vi "Main Page.vi"(8 "error in (no error)":errorcluster, 11 "Node Ptr":T7 format="%.0x") -> (0 "error out":errorcluster)   [LabVIEW 2020, in "Modbus Master System Explorer.lvlib"]
uses:
  Modbus Master System Explorer.lvlib
  <vilib>/NI VeriStand/Custom Device API/Custom Device Item Ref.ctl
  Shared/Controls/Interface Type.ctl
  Shared/Controls/Parity.ctl
  Shared/Controls/Serial Type.ctl
  Shared/Controls/Flow Control.ctl
  SubVIs/Radix.ctl
  Shared/Write Mode.ctl
  Shared/Constants.vi
  <vilib>/NI VeriStand/Custom Device API/Set Item Property (U16).vi
  <vilib>/NI VeriStand/Custom Device API/Custom Device API.lvlib
  Shared/Modbus Master Shared.lvlib
panel:
  out "Version":string
  in  "Write Refresh Rate (ms)":i32
  in  "Write Mode":T1
  in  "WebBrowser":refnum<k7>(container)
  in  "Maximum Channels per Read":i32
  in  "Read Refresh Rate (ms)":i32
  in  "Export to Kepware Server":bool
  in  "Name":string
  in  "Master Settings Tabs":enum32{"TCP Master", "Serial Master"}(tab)
  in  "Timeout (ms)":i32
  in  "Address":string
  in  "Port":u16
  in  "Baud Rate":string(combo)
  in  "Radix":T2
  in  "Unit ID":u16
  out "Data Bits":u32=7
  in  "VISA resource name":refnum<visa-resource-name>
  in  "flow control (none)":T3 items=["None", "XON/XOFF", "RTS/CTS", "XON/XOFF & RTS/CTS", "DTR/DSR", "XON/XOFF & DTR/DSR"]
  in  "parity (even)":T4=2 items=["None", "Odd", "Even", "Mark", "Space"]
  in  "serial type":T5
  out "Stop Bits":u32
  in  "Wire Mode":i16(ring)=-1 items=["Unknown"=-1, "RS485/Wire4"=0, "RS485/Wire2-EchoDTR"=1, "RS485/Wire2-CtrlDTR"=2, "RS485/Wire2-Auto"=3, "RS232/DTE"=128, "RS232/DCE"=129, "RS232/AUTO"=130]
  in  "Interface Type":T6
  in  "Header":cluster{"Section Name":string}={"Section Name"="Modbus Master to Slave Settings"}
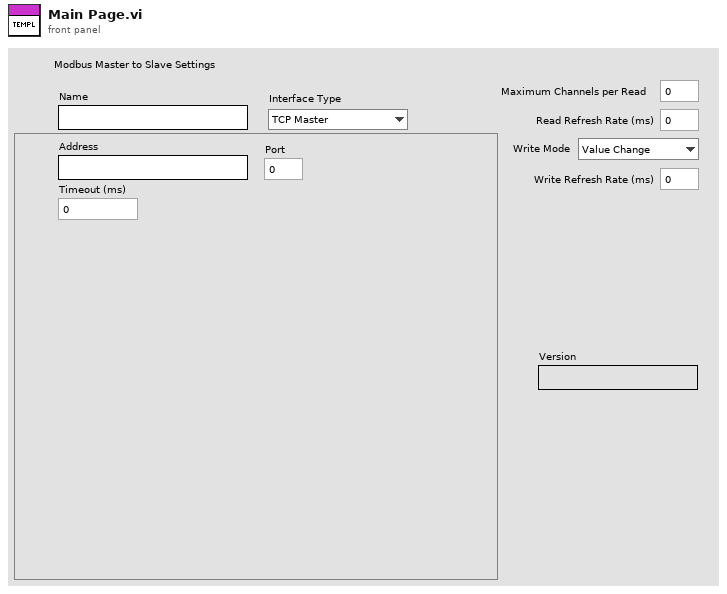
[diagram p1: front panel]
types:
  T1 = typedef "Modbus Master Shared.lvlib/Write Mode.ctl" = enum16{"Value Change", "Interval"}
  T2 = typedef "Modbus Master System Explorer.lvlib/Radix.ctl" = enum32{"Decimal", "Hexidecimal"}
  T3 = typedef "Modbus Master Shared.lvlib/Flow Control.ctl" = u16
  T4 = typedef "Modbus Master Shared.lvlib/Parity.ctl" = u16
  T5 = typedef "Modbus Master Shared.lvlib/Serial Type.ctl" = enum16{"RTU", "ASCII"}
  T6 = typedef "Modbus Master Shared.lvlib/Interface Type.ctl" = enum16{"TCP Master", "Serial Master", "TCP Slave", "Serial Slave"}
  T7 = typedef "Custom Device API.lvlib/Custom Device Item Ref.ctl" = u64
  T8 = enum8{"Enabled", "Disabled", "Disabled and Grayed Out"}
  T9 = typedef "Custom Device API.lvlib/Custom Device Commands.ctl" = enum16{"Default", "Item renamed", "Shutdown", "Dynamic button pressed"}
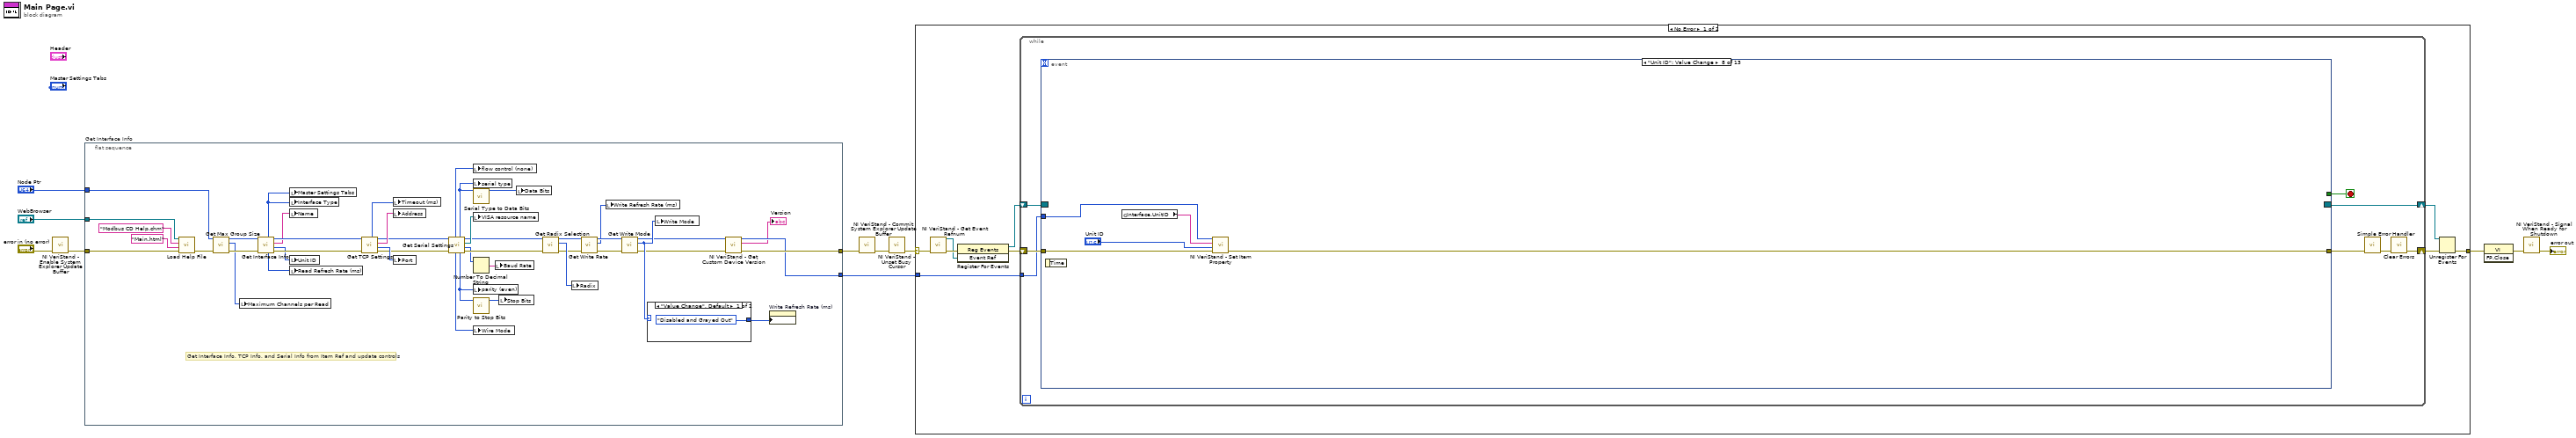
[diagram p0: block diagram]
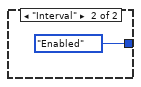
[diagram p2: hidden frame]
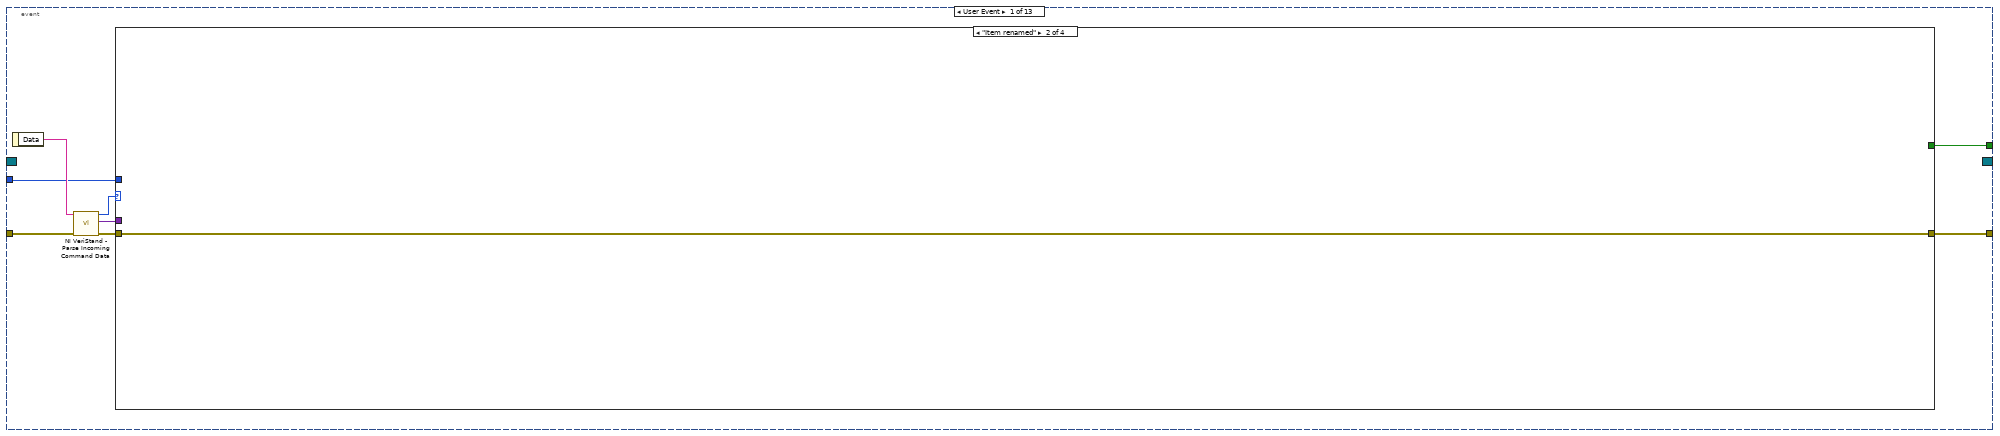
[diagram p3: hidden frame]
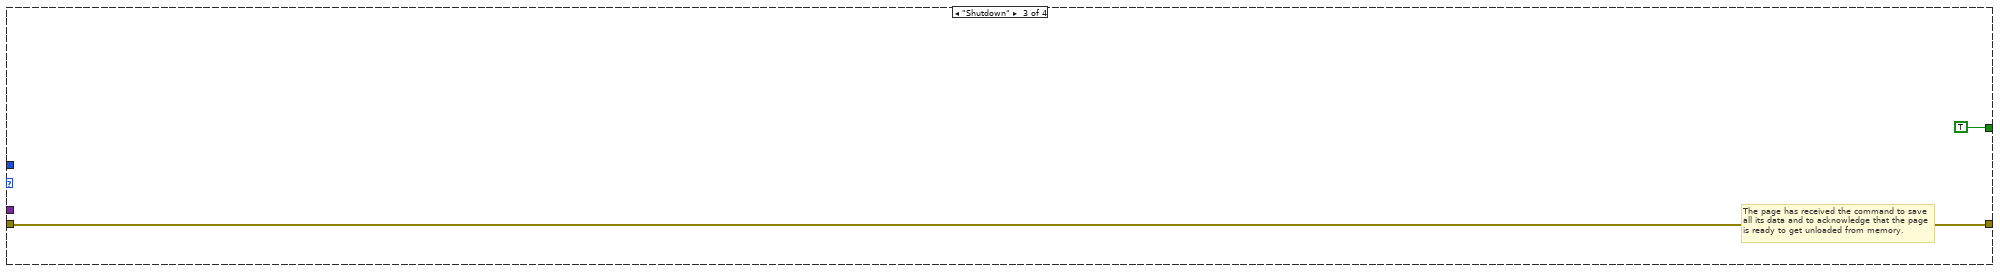
[diagram p5: hidden frame]
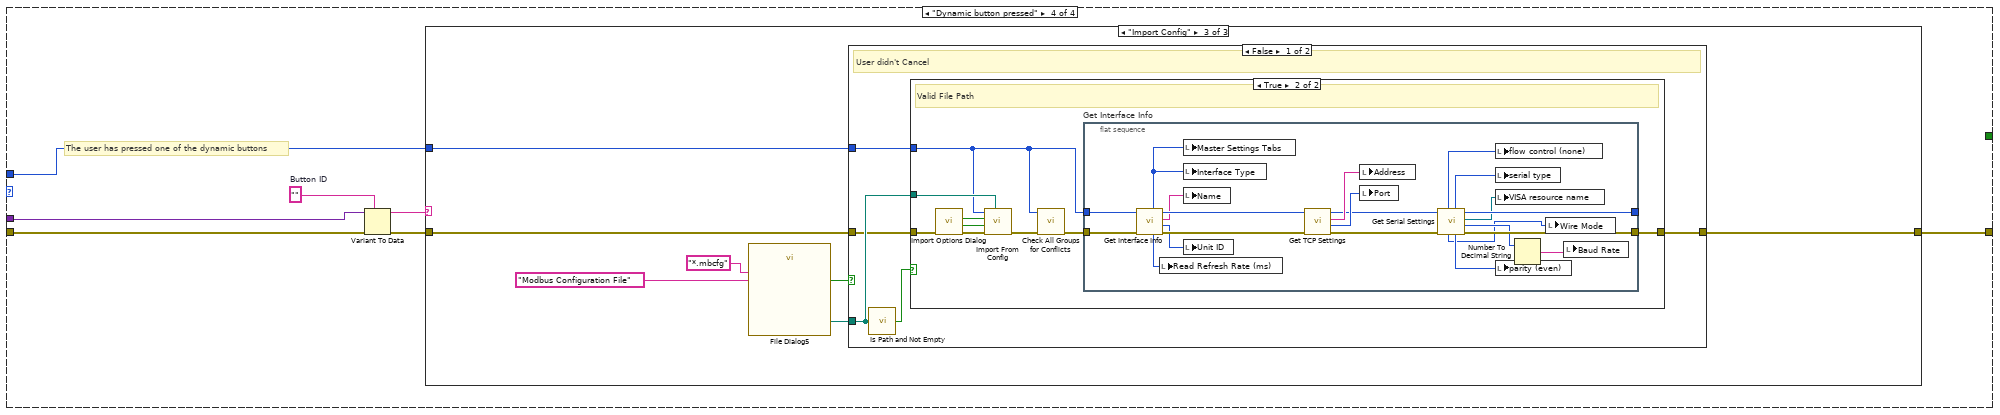
[diagram p6: hidden frame]
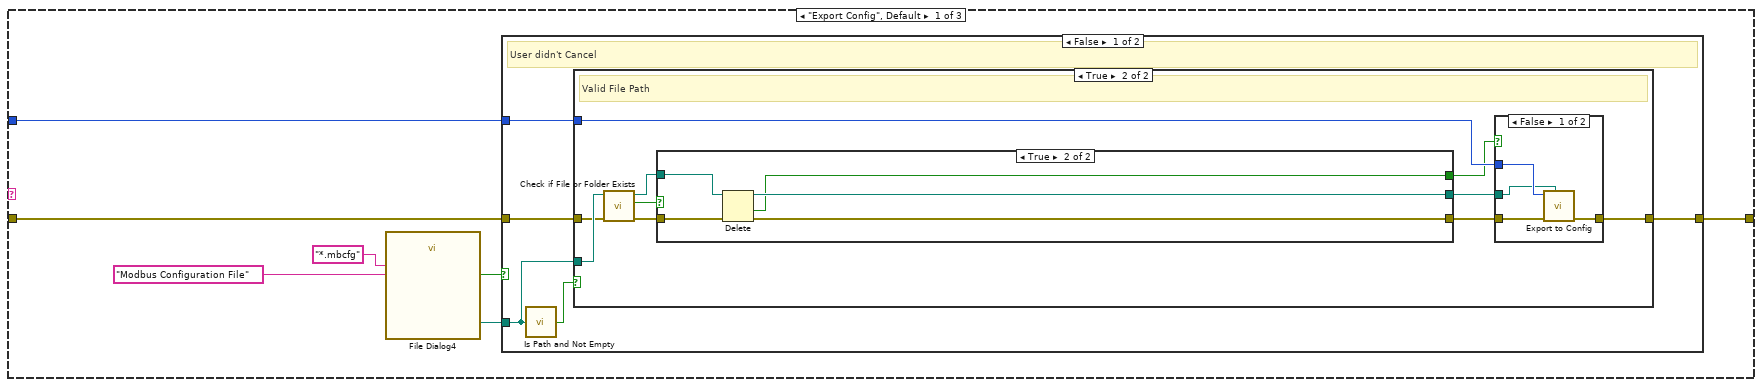
[diagram p7: hidden frame]
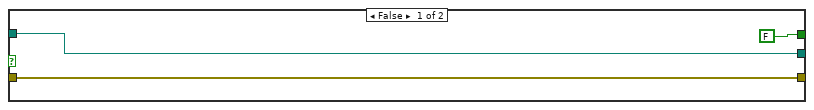
[diagram p9: hidden frame]
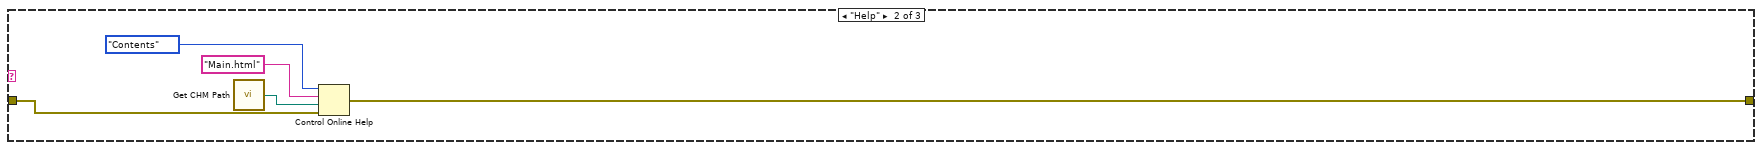
[diagram p12: hidden frame]
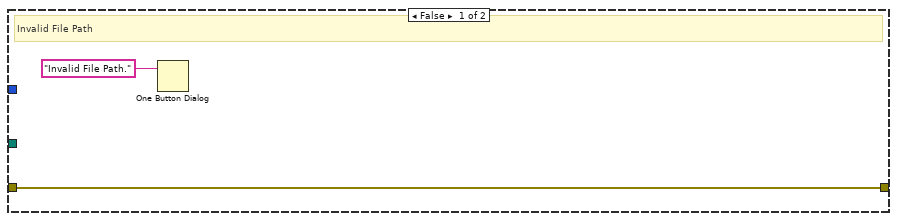
[diagram p13: hidden frame]
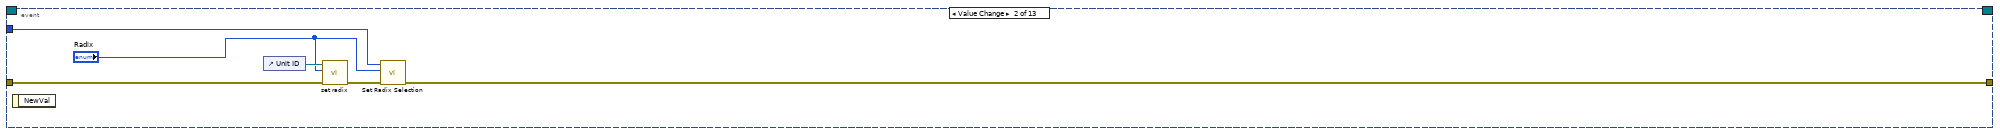
[diagram p15: hidden frame]
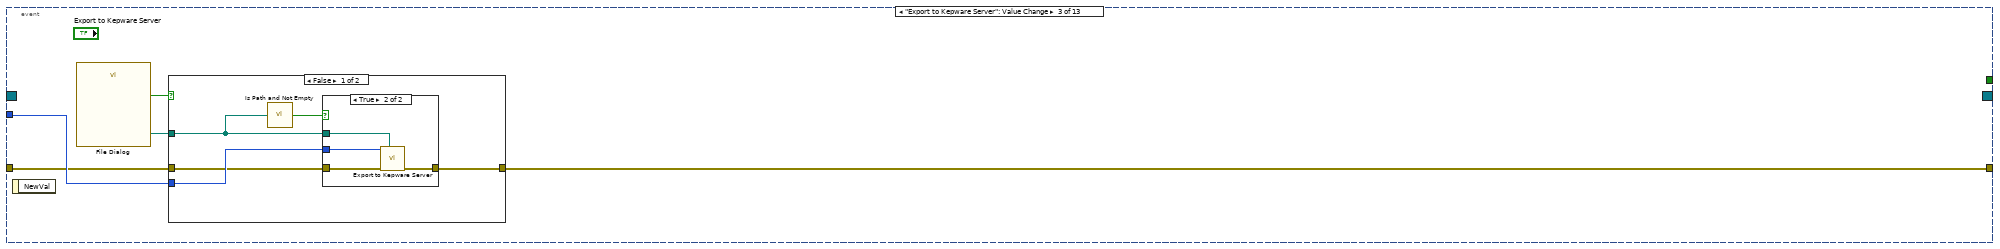
[diagram p16: hidden frame]
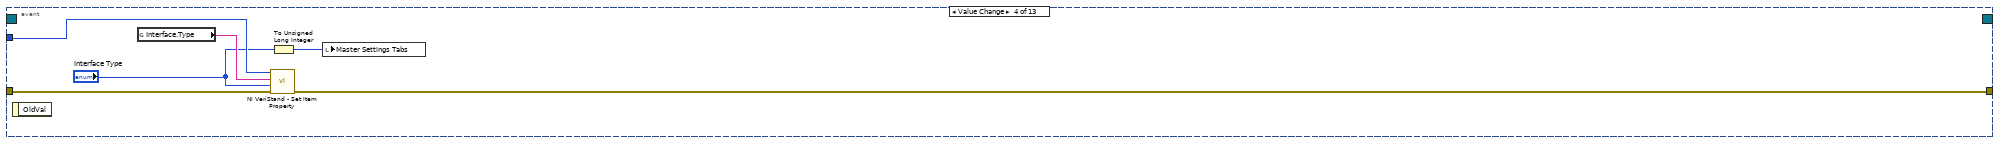
[diagram p19: hidden frame]
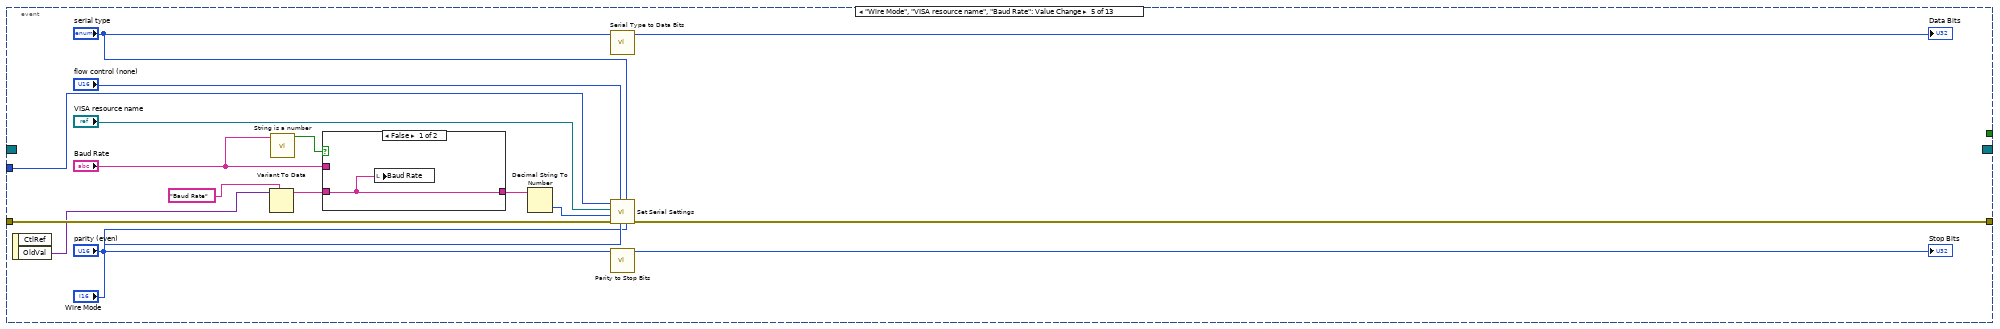
[diagram p20: hidden frame]
diagram:
  n1 = call <vilib>:"NI VeriStand - Enable System Explorer Update Buffer.vi"("error in (no error)"="error in (no error)") -> ("error out"=w1:errorcluster)  [unwired: 10 in]
  n2 = flat-sequence "Get Interface Info" {
    tunnel: w1 -> [w26]
    tunnel: "Node Ptr" -> [w39]
    tunnel: [w15] -> w4
    tunnel: [w13] -> w6
    tunnel: "WebBrowser" -> [w29]
    frame #0 {
      # "Get Interface Info, TCP Info, and Serial Info from Item Ref and update controls"
      n3 = call "Load Help File.vi"("error in (no error)"=w26, "HTML File"="Main.html", "Main CHM File"="Modbus CD Help.chm", "SHDocVw.IWebBrowser2"=w29) -> ("error out"=w25:errorcluster)  [unwired: 7 in]
      n4 = call "Get Max Group Size.vi"("error in (no error)"=w25, "Item Ref in"=w39) -> ("error out"=w37:errorcluster, "Value"=w36:i32, "Item Ref out"=w38:T7)  [unwired: 7 in]
      n5 = local write "Maximum Channels per Read"(w36) -> ()
      n6 = call "Get Interface Info.vi"("error in (no error)"=w37, "Device Item Ref in"=w38) -> ("error out"=w48:errorcluster, "Unit ID"=w45:u16, "Name"=w46:string, "Item Ref out"=w49:T7, "Refresh Rate"=w44:i32, "Interface Type"=w47:T6)  [unwired: 4 in]
      n7 = local write "Master Settings Tabs"(w47) -> ()
      n8 = local write "Interface Type"(w47) -> ()
      n9 = local write "Name"(w46) -> ()
      n10 = local write "Unit ID"(w45) -> ()
      n11 = local write "Read Refresh Rate (ms)"(w44) -> ()
      n12 = call "Get TCP Settings.vi"("error in (no error)"=w48, "Item Ref in"=w49) -> ("error out"=w53:errorcluster, "Port"=w54:u16, "Address"=w55:string, "Item Ref out"=w52:T7, "Timeout"=w35:i32)  [unwired: 5 in]
      n13 = local write "Timeout (ms)"(w35) -> ()
      n14 = local write "Address"(w55) -> ()
      n15 = local write "Port"(w54) -> ()
      n16 = call "Get Serial Settings.vi"("error in (no error)"=w53, "Item Ref in"=w52) -> ("error out"=w34:errorcluster, "baud rate"=w31:u32, "VISA resource name"=w50:refnum<visa-resource-name>, "Item Ref out"=w33:T7, "parity (even)"=w41:T4, "serial type"=w42:T5, "Wire Mode"=w24:i32, "flow control (none)"=w51:T3)  [unwired: 2 in]
      n17 = local write "flow control (none)"(w51) -> ()
      n18 = local write "serial type"(w42) -> ()
      n19 = call "Serial Type to Data Bits.vi"("serial type"=w42) -> ("Data Bits"=w43:u32)  [unwired: 10 in]
      n20 = local write "VISA resource name"(w50) -> ()
      n21 = Number To Decimal String(number=w31) -> (decimal integer string=w30:string)  [unwired: 1 in]
      n22 = local write "parity (even)"(w41) -> ()
      n23 = call "Parity to Stop Bits.vi"("parity"=w41) -> ("Stop Bits"=w40:u32)  [unwired: 10 in]
      n24 = local write "Wire Mode"(w24) -> ()
      n25 = local write "Baud Rate"(w30) -> ()
      n26 = local write "Stop Bits"(w40) -> ()
      n27 = local write "Data Bits"(w43) -> ()
      n28 = call "Get Radix Selection.vi"("error in (no error)"=w34, "Item Ref in"=w33) -> ("error out"=w23:errorcluster, "Radix"=w32:T2, "Item Ref out"=w21:T7)  [unwired: 7 in]
      n29 = local write "Radix"(w32) -> ()
      n30 = call "Get Write Rate.vi"("error in (no error)"=w23, "Item Ref in"=w21) -> ("error out"=w22:errorcluster, "Value"=w19:i32, "Item Ref out"=w20:T7)  [unwired: 7 in]
      n31 = local write "Write Refresh Rate (ms)"(w19) -> ()
      n32 = call "Get Write Mode.vi"("error in (no error)"=w22, "Item Ref in"=w20) -> ("error out"=w16:errorcluster, "Write Mode"=w17:T1, "Item Ref out"=w14:T7)  [unwired: 7 in]
      n33 = case shown="\"Value Change\", Default" w17 {
        tunnel: [T8."Disabled and Grayed Out" ("Disabled") T8."Enabled" ("Disabled")] -> w18
        frame "Value Change", Default {
        }
        frame "Interval" {
        }
      }
      n34 = local write "Write Mode"(w17) -> ()
      n35 = call <vilib>:"NI VeriStand - Get Custom Device Version.vi"("error in (no error)"=w16, "Device Ref in"=w14) -> ("error out"=w15:errorcluster, "Value"=→"Version":string, "Device Ref out"=w13:T7)  [unwired: 7 in]
      n36 = property on="Write Refresh Rate (ms)" class="DigNum (strict)"("DisabledEnum"=w18) -> ()  [unwired: 2 in, 2 out]
    }
  }
  n37 = call <vilib>:"NI VeriStand - Commit System Explorer Update Buffer.vi"("error in (no error)"=w4) -> ("error out"=w3:errorcluster)  [unwired: 10 in]
  n38 = call <vilib>:"NI VeriStand - Unset Busy Cursor.vi"("error in (no error)"=w3) -> ("error out"=w7:errorcluster)  [unwired: 10 out]
  n39 = case shown="No Error" w7 {
    selector: w7 -> [w58 w261]
    tunnel: [w63 w259] -> w11
    tunnel: w6 -> [w59 _]
    frame No Error {
      n40 = call <vilib>:"NI VeriStand - Get Event Refnum.vi"("error in (no error)"=w58) -> ("error out"=w66:errorcluster, "Event Ref"=w62:refnum<user-event>)  [unwired: 9 out]
      n41 = register-events(error in=w66, w62) -> (reference out=w60:refnum<event-registration>, error out=w61:errorcluster)  [unwired: 1 in]
      n42 = while {
        tunnel: w59 -> [w70]
        shift-right: [w67] -> w64
        shift-left: w61 -> [w73]
        shift-right: [w74] -> w65
        shift-left: w60 -> [w72]
        stop <- w71 stop-if-true
        n43 = event shown="[7] \"Unit ID\": Value Change" {
          selector: w72 -> [_ _ _ _ _ _ _ _ _ _ _ _ _]
          dyn-events: [_ _ _ _ _ _ _ _ _ _ _ _ _] -> w74
          timeout: _ -> [_ _ _ _ _ _ _ _ _ _ _ _ _]
          tunnel: w73 -> [w82 w184 w188 w206 w223 w228 w232 w236 w242 w247 w251 w257 _]
          tunnel: [w78 _ _ _ _ _ _ _ _ _ _ _ _] -> w71
          tunnel: [w77 w182 w187 w203 w221 _ w231 w235 _ _ w250 w256 _] -> w69
          tunnel: w70 -> [w76 w186 w189 w207 w224 w230 w234 w237 w243 w248 w252 w258 _]
          event User Event {
            n44 = event-data() -> ("Data"=w81:string)  [unwired: 1 out]
            n45 = call <vilib>:"NI VeriStand - Parse Incoming Command Data.vi"("error in (no error)"=w82, "Incoming data"=w81) -> ("error out"=w80:errorcluster, "Outgoing data"=w75:variant, "Action"=w79:T9)  [unwired: 7 out]
            n46 = case shown="\"Item renamed\"" w79 {
              tunnel: w80 -> [w83 w84 w85 w93]
              tunnel: [_ _ TRUE _] -> w78
              tunnel: [w83 w84 w85 w87] -> w77
              tunnel: w76 -> [_ _ _ w89]
              tunnel: w75 -> [_ _ _ w92]
              frame "Default", Default {
              }
              frame "Item renamed" {
              }
              frame "Shutdown" {
                # "The page has received the command to save all its data and to acknowledge that the page is ready to get unloaded from memory."
              }
              frame "Dynamic button pressed" {
                w91 = ""  # Button ID
                # "The user has pressed one of the dynamic buttons"
                n47 = Variant To Data(error in=w93, type=w91, Variant=w92) -> (data=w90:string, error out=w88:errorcluster)
                n48 = case shown="\"Import Config\"" w90 {
                  tunnel: w89 -> [w98 _ w140]
                  tunnel: w88 -> [w97 w132 w139]
                  tunnel: [w96 w131 w138] -> w87
                  frame "Export Config", Default {
                    n49 = call "File Dialog4"("pattern (all files)"="*.mbcfg", "pattern label"="Modbus Configuration File") -> ("selected path"=w100:path, "cancelled"=w99:bool)  [unwired: 10 in, 2 out]
                    n50 = case shown="False" w99 {
                      tunnel: w100 -> [w104 _]
                      tunnel: w98 -> [w103 _]
                      tunnel: w97 -> [w102 w130]
                      tunnel: [w101 w130] -> w96
                      frame False {
                        # "User didn't Cancel"
                        n51 = call <vilib>:"Is Path and Not Empty.vi"("path"=w104) -> ("Is Path and Not Empty?"=w105:bool)  [unwired: 4 in]
                        n52 = case shown="True" w105 {
                          tunnel: w104 -> [_ w111]
                          tunnel: w103 -> [_ w115]
                          tunnel: w102 -> [w106 w108]
                          tunnel: [w106 w116] -> w101
                          frame False {
                          }
                          frame True {
                            # "Valid File Path"
                            n53 = call <vilib>:"Check if File or Folder Exists.vi"("error in (no error)"=w108, "path"=w111) -> ("error out"=w107:errorcluster, "file or folder exists?"=w109:bool, "dup path"=w110:path)  [unwired: 7 in]
                            n54 = case shown="True" w109 {
                              tunnel: [w119 w124] -> w114
                              tunnel: [FALSE ("cancelled") w123] -> w113
                              tunnel: w107 -> [w118 w122]
                              tunnel: [w118 w121] -> w112
                              tunnel: w110 -> [w119 w120]
                              frame False {
                              }
                              frame True {
                                n55 = Delete(path (use dialog)=w120, error in=w122) -> (deleted path=w124:path, cancelled=w123:bool, error out=w121:errorcluster)  [unwired: 3 in]
                              }
                            }
                            n56 = case shown="False" w113 {
                              tunnel: w112 -> [w128 w129]
                              tunnel: [w127 w129] -> w116
                              tunnel: w115 -> [w126 _]
                              tunnel: w114 -> [w125 _]
                              frame False {
                                n57 = call "Export to Config.vi"("selected path"=w125, "error in"=w128, "Device Ref in"=w126) -> ("error out"=w127:errorcluster)  [unwired: 8 in]
                              }
                              frame True {
                              }
                            }
                          }
                        }
                      }
                      frame True {
                      }
                    }
                  }
                  frame "Help" {
                    n58 = call "Get CHM Path.vi"() -> ("appended path"=w135:path)
                    n59 = Control Online Help(1:w132, 2:w135, 3:"Main.html" ("String to search for"), 4:enum16{"Contents", "Key", "Close"}."Contents" ("Operation")) -> (0:w131:errorcluster)
                  }
                  frame "Import Config" {
                    n60 = call "File Dialog5"("pattern (all files)"="*.mbcfg", "pattern label"="Modbus Configuration File") -> ("selected path"=w142:path, "cancelled"=w141:bool)  [unwired: 10 in, 2 out]
                    n61 = case shown="False" w141 {
                      tunnel: w142 -> [w146 _]
                      tunnel: w140 -> [w145 _]
                      tunnel: w139 -> [w144 w180]
                      tunnel: [w143 w180] -> w138
                      frame False {
                        # "User didn't Cancel"
                        n62 = call <vilib>:"Is Path and Not Empty.vi"("path"=w146) -> ("Is Path and Not Empty?"=w147:bool)  [unwired: 4 in]
                        n63 = case shown="True" w147 {
                          tunnel: w146 -> [_ w158]
                          tunnel: w145 -> [_ w156]
                          tunnel: w144 -> [w149 w153]
                          tunnel: [w149 w154] -> w143
                          frame False {
                            # "Invalid File Path"
                            n64 = One Button Dialog(message="Invalid File Path.") -> ()  [unwired: 1 in, 1 out]
                          }
                          frame True {
                            # "Valid File Path"
                            n65 = call "Import Options Dialog.vi"("error in (no error)"=w153) -> ("error out"=w152:errorcluster, "Overwrite Existing Channels?"=w150:bool, "Overwrite Device Settings?"=w151:bool)  [unwired: 8 in]
                            n66 = call "Import From Config.vi"("selected path"=w158, "error in"=w152, "Overwrite Existing Channels?"=w150, "Overwrite Device Settings?"=w151, "Device Ref in"=w156) -> ("error out"=w157:errorcluster)  [unwired: 6 in]
                            n67 = call "Check All Groups for Conflicts.vi"("error in (no error)"=w157, "Item Ref in"=w156) -> ("error out"=w155:errorcluster)  [unwired: 9 in]
                            n68 = flat-sequence "Get Interface Info" {
                              tunnel: w155 -> [w162]
                              tunnel: w156 -> [w163]
                              tunnel: [w176] -> w154
                              tunnel: [w174] -> _
                              frame #0 {
                                n69 = call "Get Interface Info.vi"("error in (no error)"=w162, "Device Item Ref in"=w163) -> ("error out"=w168:errorcluster, "Unit ID"=w165:u16, "Name"=w166:string, "Item Ref out"=w169:T7, "Refresh Rate"=w164:i32, "Interface Type"=w167:T6)  [unwired: 4 in]
                                n70 = local write "Read Refresh Rate (ms)"(w164) -> ()
                                n71 = local write "Master Settings Tabs"(w167) -> ()
                                n72 = local write "Interface Type"(w167) -> ()
                                n73 = local write "Name"(w166) -> ()
                                n74 = local write "Unit ID"(w165) -> ()
                                n75 = call "Get TCP Settings.vi"("error in (no error)"=w168, "Item Ref in"=w169) -> ("error out"=w177:errorcluster, "Port"=w178:u16, "Address"=w179:string, "Item Ref out"=w175:T7)  [unwired: 5 in, 1 out]
                                n76 = local write "Address"(w179) -> ()
                                n77 = local write "Port"(w178) -> ()
                                n78 = call "Get Serial Settings.vi"("error in (no error)"=w177, "Item Ref in"=w175) -> ("error out"=w176:errorcluster, "baud rate"=w161:u32, "VISA resource name"=w170:refnum<visa-resource-name>, "Item Ref out"=w174:T7, "parity (even)"=w173:T4, "serial type"=w172:T5, "Wire Mode"=w159:i32, "flow control (none)"=w171:T3)  [unwired: 2 in]
                                n79 = local write "flow control (none)"(w171) -> ()
                                n80 = local write "serial type"(w172) -> ()
                                n81 = local write "VISA resource name"(w170) -> ()
                                n82 = local write "parity (even)"(w173) -> ()
                                n83 = Number To Decimal String(number=w161) -> (decimal integer string=w160:string)  [unwired: 1 in]
                                n84 = local write "Wire Mode"(w159) -> ()
                                n85 = local write "Baud Rate"(w160) -> ()
                              }
                            }
                          }
                        }
                      }
                      frame True {
                        # "User Canecelled, do nothing"
                      }
                    }
                  }
                }
              }
            }
          }
          event Value Change {
            n86 = event-data() -> ()  [unwired: 2 out]
            n87 = control-ref of="Unit ID"() -> (w185:refnum<vi>)
            n88 = call "set radix.vi"("error in (no error)"=w184, "Radix"="Radix", "Digital in"=w185) -> ("error out"=w183:errorcluster)  [unwired: 8 in]
            n89 = call "Set Radix Selection.vi"("error in (no error)"=w183, "Radix"="Radix", "Item Ref in"=w186) -> ("error out"=w182:errorcluster)  [unwired: 7 in, 1 out]
          }
          event "Export to Kepware Server": Value Change {
            n90 = event-data() -> ()  [unwired: 2 out]
            n91 = call "File Dialog"() -> ("selected path"=w191:path, "cancelled"=w190:bool)  [unwired: 12 in, 2 out]
            n92 = case shown="False" w190 {
              tunnel: w191 -> [w195 _]
              tunnel: w189 -> [w194 _]
              tunnel: w188 -> [w193 w202]
              tunnel: [w192 w202] -> w187
              frame False {
                n93 = call <vilib>:"Is Path and Not Empty.vi"("path"=w195) -> ("Is Path and Not Empty?"=w196:bool)  [unwired: 4 in]
                n94 = case shown="True" w196 {
                  tunnel: w195 -> [_ w201]
                  tunnel: w194 -> [_ w200]
                  tunnel: w193 -> [w197 w199]
                  tunnel: [w197 w198] -> w192
                  frame False {
                  }
                  frame True {
                    n95 = call "Export to Kepware Server.vi"("selected path"=w201, "error in"=w199, "Device Ref in"=w200) -> ("error out"=w198:errorcluster)  [unwired: 8 in]
                  }
                }
              }
              frame True {
              }
            }
          }
          event Value Change {
            n96 = event-data() -> ()  [unwired: 2 out]
            n97 = global read "Constants.vi" "Interface.Type"() -> (w208:string)
            n98 = call-poly <vilib>:"NI VeriStand - Set Item Property.vi"("error in (no error)"=w206, "Value"="Interface Type", "Property Name"=w208, "Item Ref in"=w207) -> ("error out"=w203:errorcluster)  [unwired: 5 in, 2 out]
            n99 = To Unsigned Long Integer(number="Interface Type") -> (unsigned 32bit integer=w205:u32)
            n100 = local write "Master Settings Tabs"(w205) -> ()
          }
          event "Wire Mode", "VISA resource name", "Baud Rate": Value Change {
            n101 = event-data() -> ("OldVal"=w211:variant)  [unwired: 2 out]
            n102 = Variant To Data(type="Baud Rate" ("y"), Variant=w211) -> (data=w210:string)  [unwired: 1 in, 1 out]
            n103 = call "String is a number.vi"("Baud Rate"="Baud Rate") -> ("Boolean"=w214:bool)  [unwired: 10 in]
            n104 = case shown="False" w214 {
              tunnel: "Baud Rate" -> [_ w227]
              tunnel: [w226 w227] -> w212
              tunnel: w210 -> [w226 _]
              frame False {
                n105 = local write "Baud Rate"(w226) -> ()
              }
              frame True {
              }
            }
            n106 = Decimal String To Number(string=w212) -> (number=w218:i32)  [unwired: 2 in, 1 out]
            n107 = call "Serial Type to Data Bits.vi"("serial type"="serial type") -> ("Data Bits"=→"Data Bits":u32)  [unwired: 10 in]
            n108 = call "Set Serial Settings.vi"("Wire Mode"="Wire Mode", "serial type"="serial type", "parity (even)"="parity (even)", "flow control (none)"="flow control (none)", "error in (no error)"=w223, "baud rate"=w218, "VISA resource name"="VISA resource name", "Item Ref in"=w224) -> ("error out"=w221:errorcluster)  [unwired: 2 in, 1 out]
            n109 = call "Parity to Stop Bits.vi"("parity"="parity (even)") -> ("Stop Bits"=→"Stop Bits":u32)  [unwired: 10 in]
          }
          event "Maximum Channels per Read": Value Change {
            n110 = event-data() -> ()  [unwired: 7 out]
            n111 = call "Set Max Group Size.vi"("error in (no error)"=w228, "Value"="Maximum Channels per Read", "Item Ref in"=w230) -> ()  [unwired: 7 in, 2 out]
          }
          event "Name": Value Change {
            n112 = event-data() -> ()  [unwired: 4 out]
            n113 = call "update name.vi"("error in (no error)"=w232, "Desired Alias"="Name", "Parent Ref in"=w234) -> ("error out"=w231:errorcluster)  [unwired: 7 in, 1 out]
          }
          event "Unit ID": Value Change {
            n114 = event-data() -> ()  [unwired: 2 out]
            n115 = global read "Constants.vi" "Interface.UnitID"() -> (w239:string)
            n116 = call-poly <vilib>:"NI VeriStand - Set Item Property.vi"("error in (no error)"=w236, "Value"="Unit ID", "Property Name"=w239, "Item Ref in"=w237) -> ("error out"=w235:errorcluster)  [unwired: 5 in, 2 out]
          }
          event Value Change {
            n117 = event-data() -> ()  [unwired: 7 out]
            n118 = call "Set Write Mode.vi"("error in (no error)"=w242, "Write Mode"="Write Mode", "Item Ref in"=w243) -> ()  [unwired: 7 in, 2 out]
            n119 = case shown="\"Value Change\", Default" "Write Mode" {
              tunnel: [T8."Disabled and Grayed Out" ("Disabled") T8."Enabled" ("Disabled")] -> w240
              frame "Value Change", Default {
              }
              frame "Interval" {
              }
            }
            n120 = property on="Write Refresh Rate (ms)" class="DigNum (strict)"("DisabledEnum"=w240) -> ()  [unwired: 2 in, 2 out]
          }
          event "Write Refresh Rate (ms)": Value Change {
            n121 = event-data() -> ()  [unwired: 7 out]
            n122 = call "Set Write Rate.vi"("error in (no error)"=w247, "Value"="Write Refresh Rate (ms)", "Item Ref in"=w248) -> ()  [unwired: 7 in, 2 out]
          }
          event "Read Refresh Rate (ms)": Value Change {
            n123 = event-data() -> ()  [unwired: 5 out]
            n124 = call "Set Refresh Rate.vi"("error in (no error)"=w251, "Value"="Read Refresh Rate (ms)", "Item Ref in"=w252) -> ("error out"=w250:errorcluster)  [unwired: 7 in, 1 out]
          }
          event "Address", "Port", "Timeout (ms)": Value Change {
            n125 = event-data() -> ()  [unwired: 4 out]
            n126 = call "Set TCP Settings.vi"("Timeout"="Timeout (ms)", "error in (no error)"=w257, "Port"="Port", "Address"="Address", "Item Ref in"=w258) -> ("error out"=w256:errorcluster)  [unwired: 5 in, 1 out]
          }
          event "Version": Value Change {
            n127 = event-data() -> ()  [unwired: 7 out]
          }
        }
        n128 = call <vilib>:"Simple Error Handler.vi"("error in (no error)"=w69) -> ("error out"=w68:errorcluster)  [unwired: 1 in, 7 out]
        n129 = call <vilib>:"Clear Errors.vi"("error in (no error)"=w68) -> ("error out"=w67:errorcluster)  [unwired: 1 in, 5 out]
      }
      n130 = Unregister For Events(event registration refnum=w65, error in=w64) -> (error out=w63:errorcluster)
    }
    frame Error {
      n131 = call <vilib>:"Simple Error Handler.vi"("error in (no error)"=w261) -> ("error out"=w260:errorcluster)  [unwired: 1 in, 7 out]
      n132 = call <vilib>:"Clear Errors.vi"("error in (no error)"=w260) -> ("error out"=w259:errorcluster)  [unwired: 1 in, 5 out]
    }
  }
  n133 = invoke class="VI" method="FP.Close"(error in=w11) -> (error out=w10:errorcluster)  [unwired: 2 in, 2 out]
  n134 = call <vilib>:"NI VeriStand - Signal When Ready for Shutdown.vi"("error in (no error)"=w10) -> ("error out"=→"error out":errorcluster)  [unwired: 10 out]
